vi "Open FITS Reference.vi"(8 "error in (no error)":errorcluster, 11 "Save Image in":refnum<class "Save Image.lvclass">) -> (0 "error out":errorcluster, 3 "Save Image out":refnum<class "Save Image.lvclass">)   [LabVIEW 2018, in "Save Image.lvclass"]
uses:
  Save Image.lvclass
  Save Image.lvclass/Save Image.ctl
  <userlib>/gfitsio/gfitsio.lvlib
  Simulated_Header/Simulated_Header.lvclass
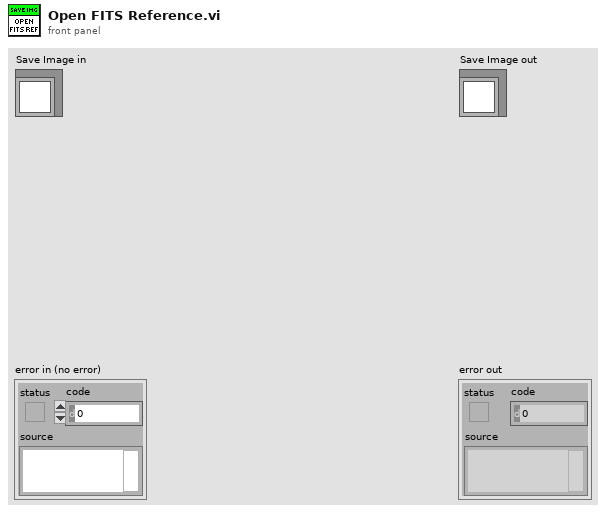
[diagram p1: front panel]
types:
  T1 = enum16{"open", "open or create", "create or replace", "create", "open (read only)"}
  T2 = cluster{"COMNENT":string, "OBSTYPE":string, "ACSVRSN":string, "CHANNEL":u16, "LAST_IMG_NAME":string, "NIGHTDIR":string}
  T3 = typedef "gfitsio.lvlib/gfitsio-refnum.ctl" = refnum<k1>
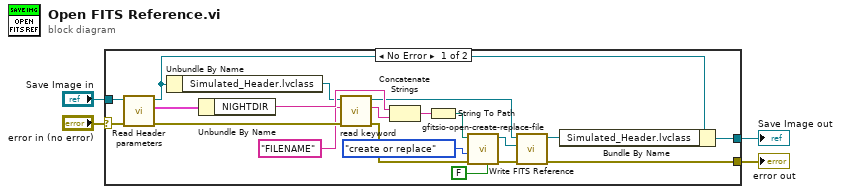
[diagram p0: block diagram]
diagram:
  n1 = case shown="No Error" "error in (no error)" {
    selector: "error in (no error)" -> [w22 w26]
    tunnel: [w19 w26] -> w3
    tunnel: [w16 w25] -> w1
    tunnel: "Save Image in" -> [w23 w25]
    frame No Error {
      n2 = call "Read Header parameters.vi"("error in (no error)"=w22, "Save Image in"=w23) -> ("error out"=w10:errorcluster, "Header parameters"=w15:T2, "Save Image out"=w17:refnum<class "Save Image.lvclass">)  [unwired: 7 in]
      n3 = Unbundle By Name(w17) -> ("Simulated_Header.lvclass"=w11:refnum<class "Simulated_Header.lvclass">)
      n4 = Unbundle By Name(w15) -> ("NIGHTDIR"=w14:string)
      n5 = call "read keyword.vi"("error in (no error)"=w10, "keyword"="FILENAME", "Simulated_Header in"=w11) -> ("error out"=w9:errorcluster, "value"=w6:string, "Simulated_Header out"=w8:refnum<class "Simulated_Header.lvclass">)  [unwired: 6 in]
      n6 = Concatenate Strings(w14, w6) -> (w13:string)
      n7 = String To Path(string=w13) -> (path=w12:path)
      n8 = call <userlib>:"gfitsio-open-create-replace-file.vi"("advisory dialog? (display:T)"=FALSE, "error in (no error)"=w9, "function (open)"=T1."create or replace", "file path (dialog if empty)"=w12) -> ("error out"=w20:errorcluster, "gfits refnum"=w21:T3)  [unwired: 5 in, 1 out]
      n9 = call "Write FITS Reference.vi"("error in (no error)"=w20, "gfits refnum"=w21, "Simulated_Header in"=w8) -> ("error out"=w19:errorcluster, "Simulated_Header out"=w18:refnum<class "Simulated_Header.lvclass">)  [unwired: 7 in]
      n10 = Bundle By Name(cluster=w17, "Simulated_Header.lvclass"=w18) -> (w16:refnum<class "Save Image.lvclass">)
    }
    frame Error {
    }
  }
  "error out" <- w3
  "Save Image out" <- w1
